vi "PS-OCTA-OCE-autofocus.vi"() -> ()   [LabVIEW 2024] (continued)
  T20 = cluster{"AcqCursorList":T9, "RecalFringePhaseFit_Inv":dbl[][], "RawDualBackgroundArray":i16[][], "RawSingleBackgroundArray":i16[][], "RawRecalFringeArray":i16[][], "RecalFringePhaseFit":dbl[][], "SingleBackground":i16[], "DualBackground":i16[], "image crop start":i32, "cut_level_low":dbl, "cut_level_high":dbl, "Raw1mmFringeArray":i16[][], "img_bckg_offset":i32, "img_bckg_length":i32, "DVV":i16[][], "DVV_shift":i32, "disp_coef":dbl}[]
  T21 = typedef "imagedata.ctl" = cluster{"image type":i32, "image depth":i32, "image":u8[], "mask":u8[], "colors":u32[], "Rectangle":cluster{"left":i16, "top":i16, "right":i16, "bottom":i16}}
  T22 = cluster{"n_f to c. trig":i32, "c. trig length":i32, "c. trig interval":i32, "n_c. trig":i32}
  T23 = cluster{dbl, i32, "cut_level_high":dbl, "cut_level_low":dbl, "offset":i32, "length":i32, "crop start":i32, i32}
  T24 = cluster{"Robot Vel":dbl, "Robot Acc":dbl, "Z-tolerance (mm)":dbl, "Angle tolerance (deg)":dbl, i32, "Radius (mm)":dbl, "Angle End (deg)":dbl, "Number of points":i32, bool, "Z height (pixel)":dbl, "X (mm)":dbl, "Y (mm) ":dbl, "Apply Offset":bool, "Angle Start (deg)":dbl, "N OCT":i32}
  T25 = cluster{"Autofocus":bool, "Freedrive":bool, "Next point":bool, "Previous point":bool, "Home":bool, "Reset":bool, "Start Full Protocol":bool, "3D preview":bool, "Robot ON/OFF":bool, "Cancel Button":bool, "scan_flip_state":bool, "Robot_control":bool, "OCT_control":bool, "OCTA_control":bool, "OCE_control":bool}
  T26 = cluster{"message":string, "angle":dbl, "circle_state":dbl, "scan_trigger":bool, "apply_config":bool, "end_state":bool, "scan_3d":bool, "full_scan":bool, "robot_mode":bool, "oct_mode":bool, "octa_mode":bool, "oce_mode":bool}
  T27 = typedef "ORS_Parameter_Cluster_v8.ctl" = cluster{"file version":u32, "data set dimension":u16, "description":string, "sampling_rate":dbl, "samples_per_line":dbl, "vert_range":dbl, "various params":string, "image samples per line":i32, "image height (crop)":i32, "CPI frequency per mm":dbl, "Peak samp pos\n1mm (Michels)":i32, "n_channel":i32, "Buffer factor":i32, "Per Channel Params":T8, "Galvo":T5, "n_bit":enum16{"8bit", "16bit"}, "timestamp":string}
  T28 = cluster{"samples/line 3d":dbl, "n_lines":i32, "cut_level_high":dbl, "cut_level_low":dbl, "offset":i32, "length":i32, "crop start":i32, "image height":i32}
diagram:
  w10 = T6 {"shutter1"="", "shutter2"="", "Galvo"={"x mirror"="", "y mirror"="", "trig out"="", "x mirror task"="", "y mirror task"="", "trig out task"="", "n_axis"=0, "params"={"n_lines"=0, "n_frames"=0, "force to zero"=FALSE, "Triggers_per_sweep"=0.0, "X center"=0.0, "X span"=0.0, "Y center"=0.0, "Y span"=0.0, "flyb.lines"=0, "n_triggers"=0, "mode"=0, "offset"=0.0, "galvo phase"=0, "span factor"=0.0, "Custom trig."={"n_f to c. trig"=0, "c. trig length"=0, "c. trig interval"=0, "n_c. trig"=0}, "f_per_pos"=0, "n_dataset"=0, "flyback fr"=0}, "acq trig out"="", "acq trig out task"="", "sample array X"=[], "sample array Y"=[], "custom trig out"="", "custom trig out task"="", "FDML-box"="", "ACQ/Galvo"=enum."ADC/FDML", "acq trig out an task"="", "acq trig out an"="", "Galvo Trig input"="", "Galvo Clk input"="", "sample array Acq trig out an"=[]}, "n_bit"=enum."16bit", "diode mon"="", "Misc_I/O"=enum."None"}  # instrument cluster
  w6 = T7 {"Data source"=enum."AlazarTec", "Sample Rate"=0.0, "n_channel"=1, "At9462 # samples"=1024, "image height (crop)"=512, "B scan offset (sps)"=0.0, "window"=0, "OCT data dir"=path "", "3d file name"="", "Description"="", "Galvo params only for file storage"={"n_lines"=0, "n_frames"=0, "force to zero"=FALSE, "Triggers_per_sweep"=0.0, "X center"=0.0, "X span"=0.0, "Y center"=0.0, "Y span"=0.0, "flyb.lines"=0, "n_triggers"=0, "mode"=0, "offset"=0.0, "galvo phase"=0, "span factor"=0.0, "Custom trig."={"n_f to c. trig"=0, "c. trig length"=0, "c. trig interval"=0, "n_c. trig"=0}, "f_per_pos"=0, "n_dataset"=0, "flyback fr"=0}, "Per Channel Params"=[{"AcqCursorList"=[], "RecalFringePhaseFit_Inv"=[], "RawDualBackgroundArray"=[], "RawSingleBackgroundArray"=[], "RawRecalFringeArray"=[], "RecalFringePhaseFit"=[], "SingleBackground"=[], "DualBackground"=[], "image crop start"=0, "cut_level_low"=70.0, "cut_level_high"=110.0, "Raw1mmFringeArray"=[], "img_bckg_offset"=0, "img_bckg_length"=20, "DVV"=[], "DVV_shift"=20, "disp_coef"=0.0}], "file version"=8, "do_dual_card"=FALSE, "ATS_clock"={"Source"=2, "Sample Rate"=48, "Edge"=0, "Rate Ext Ref"=400000000, "Trigger Delay"=100, "Rate Int Ref"=450}, "ATS_clock 2"={"Source"=8, "Sample Rate"=48, "Edge"=0, "Rate Ext Ref"=400000000, "Trigger Delay"=0, "Rate Int Ref"=500}, "DES"=FALSE, "digi_trig"=TRUE, "Ch. Select"=[TRUE, TRUE, FALSE, FALSE, FALSE, FALSE, FALSE, FALSE], "Override Ch."=[FALSE, FALSE, FALSE, FALSE, FALSE, FALSE, FALSE, FALSE], "DoInterp"=TRUE, "EnableDVV"=FALSE, "bufferCount"=128, "dispcoef"=0.0, "AO.type"=12590, "Disable Bck"=[FALSE, FALSE, FALSE, FALSE, FALSE, FALSE, FALSE, FALSE], "PhaseCompVector"=array[2304 elements], "DoDispComp"=FALSE, "Load Insight?"=FALSE, "ChannelDisp"=1, "Zoom Factor"=0.0, "FFT Down Sample"=1, "cut_level_high"=127.0, "cut_level_low"=40.0, "Channel"=3, "IgnoreBadClk"=FALSE, "Good_Clock"=2.65e-06, "Bad_Clock"=2.05e-06}  # General state cluster
  # "command array cmds"
  # "cmds"
  # "instrument cluster - instr"
  n1 = local write "Roll-off"(dbl[][] [] ("Roll-off")) -> ()
  n2 = local write "Roll-off_RawData"(i32[][] [] ("Roll-off")) -> ()
  n3 = call <vilib>:"Application Directory.vi"() -> ("Application Directory"=w4:path)
  n4 = Build Path(base path=w4, name or relative path="Custom state file") -> (appended path=w2:path)
  n5 = call "serial_read_write.vi"("Enable Delayline"="Enable Delayline", "VISA Refnum in"="VISA resource name") -> ()  [unwired: 10 in]
  n6 = Build Array("ConfigAndDisplay") -> (w12:string[])
  n7 = case shown="True" "LoadConfig?" {
    tunnel: w12 -> [w14 w15]
    tunnel: [w14 w17] -> w11
    frame False {
    }
    frame True {
      n8 = Build Array (concatenate)("LoadDefaultState", w15) -> (w17:string[])
    }
  }
  n9 = stacked-sequence {
    seq-local: [w19 _ _] -> [_ w64 w1997]
    tunnel: w6 -> [_ w63 _]
    tunnel: w11 -> [_ w62 _]
    tunnel: [_ w61 _] -> _
    tunnel: w2 -> [_ w60 _]
    tunnel: w10 -> [w21 w58 _]
    tunnel: [_ w59 _] -> _
    frame #0 {
      w18 = enum16{"8bit", "16bit"}."16bit"  # n_bit
      # "INIT\nsystem initialization"
      n10 = Bundle By Name(cluster=w21, "n_bit"=w18) -> (w20:T6)
      n11 = flat-sequence {
        tunnel: w20 -> [w40]
        tunnel: [w37] -> w19
        frame #0 {
          w23 = TRUE ("Apply Acq Config")
          w39 = "(none)" ("Time of background capture")
          # "Misc I/O for shutters & PD monitor"
          # "acq trig for ADC card + Galvo control"
          n12 = local write "exit"(FALSE ("exit")) -> ()
          n13 = local write "Start 3D scan"(FALSE) -> ()
          n14 = local write "Apply Config"(w23) -> ()
          n15 = local write "Apply Acq Config"(w23) -> ()
          n16 = case shown="\"NI_DAQ\"" "Misc_I/O" {
            tunnel: [_ w53 _] -> w42
            tunnel: [_ w52 _] -> w41
            tunnel: [_ w49 _] -> w35
            tunnel: [enum16{"FDML", "NI_DAQ", "None"}."FDML" ("Misc_I/O") enum16{"FDML", "NI_DAQ", "None"}."NI_DAQ" ("Misc_I/O") enum16{"FDML", "NI_DAQ", "None"}."None" ("Misc_I/O")] -> w33
            frame "FDML", Default {
            }
            frame "NI_DAQ" {
              n17 = Build Array("diode monitor +", "diode monitor -") -> (w45:tag[])
              n18 = call <vilib>:"DAQmx Flatten Channel String.vi"("names in"=w45) -> ("names out"=w46:string)  [unwired: 13 in, 1 out]
              n19 = call-poly <vilib>:"DAQmx Create Virtual Channel.vi"("physical channels"=w46) -> ("task out"=w49:refnum<k21>)  [unwired: 13 in, 1 out]
              n20 = call-poly <vilib>:"DAQmx Create Virtual Channel.vi"("lines"="shutter1") -> ("task out"=w53:refnum<k21>)  [unwired: 13 in, 1 out]
              n21 = call-poly <vilib>:"DAQmx Create Virtual Channel.vi"("lines"="shutter2") -> ("task out"=w52:refnum<k21>)  [unwired: 13 in, 1 out]
            }
            frame "None" {
            }
          }
          n22 = local write "Time of last RecalFringes"(w39) -> ()
          n23 = local write "Time of background capture"(w39) -> ()
          n24 = local write "OpModeTab"(enum32{"Config", "Img:Preview"}."Config" ("OpModeTab")) -> ()
          n25 = call "ORS_GalvoInit2_uw.vi"("acq trig out"=tag "Dev1/port0/line4", "custom trig out"=tag "Dev1/port0/line7", "Galvo Clk input"=tag "/Dev1/PFI0", "trig out"=tag "Dev1/port0/line2" ("trig AND out"), "y mirror"=tag "Dev1/ao1", "x mirror"=tag "Dev1/ao0") -> ("Galvo out"=w25:T5)  [unwired: 4 in, 1 out]
          n26 = Bundle By Name(cluster=w25, "ACQ/Galvo"=enum32{"ADC/FDML", "NI_DAQ", "ADC"}."NI_DAQ") -> (w36:T5)
          n27 = Bundle By Name(cluster=w40, "diode mon"=w35, "Galvo"=w36, "shutter1"=w42, "shutter2"=w41, "Misc_I/O"=w33) -> (w37:T6)
        }
      }
    }
    frame #1 {
      w57 = 0  # n_lines
      # "MAIN"
      n28 = feedback #1() -> (w55:u8[][])  [unwired: 1 in]
      n29 = while {
        shift-right: [w87] -> w61
        shift-left: w63 -> [w88]
        shift-right: [w79] -> w59
        shift-left: w64 -> [w93]
        shift-right: [w86] -> _
        shift-left: w62 -> [w68]
        tunnel: w60 -> [w85]
        shift-right: [w84] -> _
        shift-left: _ -> [w77]
        shift-right: [w83] -> _
        shift-left: w57 -> [w82]
        shift-right: [w81] -> _
        shift-left: _ -> [w80]
        shift-right: [w79] -> _
        shift-left: _ -> [w78]
        shift-right: [w76] -> _
        shift-left: _ -> [w75]
        tunnel: w58 -> [w74]
        shift-right: [w72] -> _
        shift-left: _ -> [w71]
        shift-right: [w69] -> _
        shift-left: w55 -> [w70]
        tunnel: [u8[][] []] -> w56
        shift-right: [w65] -> _
        shift-left: _ -> [w66]
        i -> [w89]
        stop <- w73 stop-if-true
        # "skip"
        # "instr"
        # "raw"
        # "state"
        # "instr"
        # "cmds"
        # "samples per line"
        # "number of lines"
        # "This is the main program loop."
        n30 = case shown="\"Img:Preview\"" "OpModeTab" {
          tunnel: w93 -> [w101 w894]
          tunnel: [w100 w871] -> w90
          tunnel: w88 -> [w99 w895]
          tunnel: [w98 w893] -> w87
          tunnel: [w97 w892] -> w79
          tunnel: w68 -> [w96 w890]
          tunnel: [w95 w891] -> w86
          tunnel: w85 -> [w94 _]
          tunnel: [_ w889] -> w84
          tunnel: w77 -> [_ w888]
          tunnel: [_ w887] -> w83
          tunnel: w82 -> [_ w886]
          tunnel: [_ w885] -> w81
          tunnel: w80 -> [_ w884]
          tunnel: w78 -> [_ w883]
          tunnel: w77 -> [_ w882]
          tunnel: [_ w881] -> w76
          tunnel: w75 -> [_ w880]
          tunnel: w74 -> [_ w879]
          tunnel: [_ w878] -> w72
          tunnel: w71 -> [_ w877]
          tunnel: w70 -> [_ w876]
          tunnel: [_ w875] -> w69
          tunnel: w66 -> [_ w874]
          tunnel: [_ w873] -> w65
          frame "Config", Default {
            # "Config Tab"
            n31 = stacked-sequence {
              seq-local: [w114 _] -> [_ w215]
              seq-local: [w110 _] -> [_ w208]
              seq-local: [w112 _] -> [_ w213]
              seq-local: [w111 _] -> [_ w210]
              tunnel: w101 -> [w103 _]
              tunnel: [w122 _] -> w100
              tunnel: w99 -> [w108 _]
              tunnel: [_ w214] -> w98
              tunnel: [_ w209] -> w97
              tunnel: w96 -> [w117 _]
              tunnel: [_ w212] -> w95
              tunnel: w94 -> [_ w211]
              frame #0 {
                n32 = Unbundle By Name(w108) -> ("Per Channel Params"=w107:T8)
                n33 = Unbundle By Name(w103) -> ("Misc_I/O"=w102:enum16{"FDML", "NI_DAQ", "None"})
                n34 = property on="GageCursorList" class="WFGraph (strict)"() -> ("CrsrList"=w105:T9)  [unwired: 2 in, 2 out]
                n35 = for {
                  tunnel: w107 -> [w137] mode=indexing
                  tunnel: [w135] -> w106 mode=indexing
                  tunnel: w105 -> [w136]
                  n36 = Bundle By Name(cluster=w137, "AcqCursorList"=w136) -> (w135:T13)
                }
                n37 = case shown="\"NI_DAQ\"" w102 {
                  tunnel: "Override shutter 1" -> [_ w130]
                  tunnel: "Override shutter 2" -> [_ w129]
                  tunnel: w103 -> [_ w128]
                  frame "FDML", Default {
                  }
                  frame "NI_DAQ" {
                    n38 = Unbundle By Name(w128) -> ("shutter2"=w132:refnum<k21>)
                    n39 = Unbundle By Name(w128) -> ("shutter1"=w134:refnum<k21>)
                    n40 = call-poly <vilib>:"DAQmx Write.vi"("task/channels in"=w134, "auto start"=TRUE, "data"=w130) -> ()  [unwired: 10 in, 3 out]
                    n41 = call-poly <vilib>:"DAQmx Write.vi"("task/channels in"=w132, "auto start"=TRUE, "data"=w129) -> ()  [unwired: 10 in, 3 out]
                  }
                }
                n42 = local read "NumCh"() -> (w104:i32)
                n43 = Bundle By Name(cluster=w108, "Per Channel Params"=w106, "n_channel"=w104) -> (w109:T7)
                n44 = Empty Array?(array=w117) -> (empty?=w118:bool)
                n45 = Not(x=w118) -> (.not. x?=w119:bool)
                n46 = Or(x="Free running", y=w119) -> (x .or. y?=w124:bool)
                n47 = Select(t=0, s=w124, f=-1) -> (s? t:f=w127:i32)
                n48 = event shown="[11] \"exit\": Mouse Down;  \"exit\": Key Down" {
                  selector: _ -> [_ _ _ _ _ _ _ _ _ _ _ _]
                  dyn-events: _ -> [_ _ _ _ _ _ _ _ _ _ _ _]
                  timeout: w127 -> [_ _ _ _ _ _ _ _ _ _ _ _]
                  tunnel: [w138 w150 w155 w161 w166 w171 w174 w179 w185 w200 w202 w205] -> w113
                  tunnel: [_ _ _ _ _ _ _ _ _ _ _ TRUE] -> w122
                  tunnel: w109 -> [w144 w151 w156 w162 w167 w172 w175 w180 w182 w194 w203 w206]
                  tunnel: [w144 w151 w156 w162 w167 w172 w175 w180 w186 w194 w203 w206] -> w110
                  tunnel: w103 -> [w143 w149 w152 w158 w163 w168 w173 w178 w184 w197 w201 w204]
                  tunnel: w117 -> [w139 w150 w154 w159 w164 w170 w174 w179 w185 w200 w202 w205]
                  tunnel: [w143 w149 w152 w158 w163 w168 w173 w178 w184 w195 w201 w204] -> w111
                  event Timeout {
                    # "Event should trigger only on timeout."
                    n49 = event-data() -> ()  [unwired: 1 in, 2 out]
                    n50 = Array Size(array=w139) -> (size(s)=w142:i32)
                    n51 = Decrement(x=w142) -> (x-1=w141:i32)
                    n52 = Index Array(array=w139, index=w141) -> (element=w140:string)
                    n53 = case shown="Default" w140 {
                      tunnel: [w145 w147] -> w138
                      tunnel: w139 -> [w145 w146]
                      frame "ConfigAndDisplay" {
                      }
                      frame Default {
                        n54 = Build Array (concatenate)(w146, "ConfigAndDisplay") -> (w147:string[])
                      }
                    }
                  }
                  event "OpModeTab": Value Change {
                    n55 = event-data() -> ()  [unwired: 1 in, 6 out]
                  }
                  event "Capture Dual Balanced Background": Mouse Down; "Capture Dual Balanced Background": Key Down {
                    n56 = event-data() -> ()  [unwired: 1 in, 5 out]
                    n57 = Build Array (concatenate)(w154, "CaptureDualBalancedBackground") -> (w155:string[])
                  }
                  event "Save state file": Key Down; "Save state file": Mouse Down {
                    w157 = TRUE ("Apply Acq Config")
                    n58 = event-data() -> ()  [unwired: 1 in, 5 out]
                    n59 = local write "Apply Acq Config"(w157) -> ()
                    n60 = local write "Apply Config"(w157) -> ()
                    n61 = Build Array (concatenate)(w159, "SaveState") -> (w161:string[])
                  }
                  event "Load state file": Key Down; "Load state file": Mouse Down {
                    n62 = event-data() -> ()  [unwired: 1 in, 5 out]
                    n63 = Build Array (concatenate)(w164, "LoadState") -> (w166:string[])
                  }
                  event "Acquire Recal Fringes with Mirror": Key Down; "Acquire Recal Fringes with Mirror": Mouse Down {
                    n64 = event-data() -> ()  [unwired: 1 in, 5 out]
                    n65 = Build Array (concatenate)(w170, "RecalFringesMirror") -> (w171:string[])
                  }
                  event "Free running": Value Change {
                    n66 = event-data() -> ()  [unwired: 1 in, 6 out]
                  }
                  event "Re-Scale Y": Value Change {
                    n67 = event-data() -> ()  [unwired: 1 in, 6 out]
                    n68 = property on="Raw captured photodiode data" class="WFGraph (strict)"("YScale.ScaleFit"=u8 1 ("Y Scale.Scale Fit")) -> ()  [unwired: 2 in, 2 out]
                    n69 = local write "Re-Scale Y"(FALSE ("Re-Scale Y")) -> ()
                  }
                  event "Reset Dual Balanced Background": Key Down; "Reset Dual Balanced Background": Mouse Down {
                    n70 = event-data() -> ()  [unwired: 1 in, 5 out]
                    n71 = Unbundle By Name(w182) -> ("Per Channel Params"=w183:T8)
                    n72 = for {
                      tunnel: w183 -> [w187] mode=indexing
                      tunnel: [w188] -> w181 mode=indexing
                      n73 = Unbundle By Name(w187) -> ("DualBackground"=w191:i16[])
                      n74 = Multiply(x=0 ("y"), y=w191) -> (x*y=w190:i32[])
                      n75 = Bundle By Name(cluster=w187, "DualBackground"=w190) -> (w188:T13)
                    }
                    n76 = Bundle By Name(cluster=w182, "Per Channel Params"=w181) -> (w186:T7)
                  }
                  event "XY: Force zero": Value Change {
                    n77 = event-data() -> ("NewVal"=w199:bool)  [unwired: 1 in, 5 out]
                    n78 = local read "digi_trig"() -> (w193:bool)
                    n79 = local read "AO.type"() -> (w192:i32)
                    n80 = Unbundle By Name(w197) -> ("Galvo"=w198:T5)
                    n81 = call "ORS_GalvoForceToZero_uw.vi"("AO.DataXferMech"=w192, "use_digi_trig"=w193, "force to zero"=w199, "Galvo"=w198) -> ("Galvo out"=w196:T5)  [unwired: 6 in, 1 out]
                    n82 = Bundle By Name(cluster=w197, "Galvo"=w196) -> (w195:T6)
                  }
                  event "Override shutter 1", "Override shutter 2": Key Up; "Override shutter 1", "Override shutter 2": Mouse Up {
                    n83 = event-data() -> ()  [unwired: 1 in, 5 out]
                  }
                  event "exit": Mouse Down; "exit": Key Down {
                    # "Event should trigger only on ext."
                    n84 = event-data() -> ()  [unwired: 1 in, 5 out]
                  }
                }
                n85 = Split 1D Array(array=w113, index=1) -> (first subarray=w115:string[], second subarray=w112:string[])
                n86 = Index Array(array=w115) -> (element=w114:string)  [unwired: 1 in]
                "cmd list" <- w117
              }
              frame #1 {
                n87 = case shown="\"1mmFringes\", \"RecalFringes\", \"RecalFringesMirror\"" w215 {
                  selector: w215 -> [_ _ _ _ _ w599]
                  tunnel: w210 -> [w216 w223 w267 w314 w533 w602]
                  tunnel: w208 -> [w218 w224 w263 w309 w523 w601]
                  tunnel: [w218 w224 w239 w311 w524 w600] -> w214
                  tunnel: w213 -> [w217 w225 w268 w313 w529 w597]
                  tunnel: [w217 w225 w268 w312 w530 w598] -> w212
                  tunnel: w211 -> [_ w222 w257 _ _ _]
                  tunnel: [w216 w223 w266 w310 w526 w596] -> w209
                  frame "None", Default {
                    # "This case intentionally does nothing."
                  }
                  frame "SaveState" {
                    n88 = control-ref of="3D_Galvo_Params"() -> (w221:refnum<vi>)
                    n89 = control-ref of="Data Valid Vector"() -> (w220:refnum<vi>)
                    n90 = control-ref of="Save state file"() -> (w219:refnum<vi>)
                    n91 = call "config_save_state.vi"("appended path"=w222, "General state cluster"=w224, "reference 3"=w219, "reference in"=w220, "Cluster in"=w221) -> ()  [unwired: 7 in]
                  }
                  frame "LoadDefaultState", "LoadState" {
                    w260 = T9 [{"Name"="img start", "Color"=16776960, "Style"=8, "Point Style"=13, "Name Visible"=FALSE, "Allow Drag"=TRUE, "Cursor Mode"=0, "Plot"=0, "Index"=0, "Position"={"X"=0.0, "Y"=0.0}, "X Scale"=0, "Y Scale"=0, "Watch Plots"=[], "Watch All Plots"=FALSE, "Plot Area"=0, "Label Offset"={"X"=0.0, "Y"=2937.5}}, {"Name"="img stop", "Color"=16776960, "Style"=8, "Point Style"=13, "Name Visible"=FALSE, "Allow Drag"=TRUE, "Cursor Mode"=0, "Plot"=0, "Index"=0, "Position"={"X"=1000.0, "Y"=0.0}, "X Scale"=0, "Y Scale"=0, "Watch Plots"=[], "Watch All Plots"=FALSE, "Plot Area"=0, "Label Offset"={"X"=3.6556291390728575, "Y"=2937.5}}, {"Name"="recal start", "Color"=16711680, "Style"=8, "Point Style"=13, "Name Visible"=FALSE, "Allow Drag"=TRUE, "Cursor Mode"=0, "Plot"=0, "Index"=0, "Position"={"X"=108.50331125827815, "Y"=0.0}, "X Scale"=0, "Y Scale"=0, "Watch Plots"=[], "Watch All Plots"=FALSE, "Plot Area"=0, "Label Offset"={"X"=0.0, "Y"=2937.5}}, {"Name"="recal stop", "Color"=16711680, "Style"=8, "Point Style"=13, "Name Visible"=FALSE, "Allow Drag"=TRUE, "Cursor Mode"=0, "Plot"=0, "Index"=0, "Position"={"X"=922.2781456953643, "Y"=0.0}, "X Scale"=0, "Y Scale"=0, "Watch Plots"=[], "Watch All Plots"=FALSE, "Plot Area"=0, "Label Offset"={"X"=0.0, "Y"=2937.5}}]  # AcqCursorList_default
                    w280 = T14 4 items=["no dialog", "OK message", "continue or stop message", "OK message + warnings", "continue/stop + warnings"] ("type of dialog (OK msg:1)")
                    # "n_lines is either #lines preview or #lines2d/3d, depending on which one has been last used\n(same for Y span and  Y center, but in almost all cases 2d should have been used before exit)"
                    n92 = local write "Load state file"(FALSE ("Save state file 2")) -> ()
                    n93 = Read from Binary File(5:w263, 9:T10."little-endian" ("byte order (0:big-endian, network order)"), 11:w257) -> (0:w279:errorcluster, 2:w262:T7)  [unwired: 3 in, 2 out]
                    n94 = call <vilib>:"General Error Handler.vi"("type of dialog (OK msg:1)"=w280, "error in (no error)"=w279) -> ("error?"=w264:bool)  [unwired: 9 in, 4 out]
                    n95 = Select(t=w263, s=w264, f=w262) -> (s? t:f=w239:T7)
                    n96 = Unbundle By Name(w239) -> ("Galvo params only for file storage"=w226:T4, "Per Channel Params"=w276:T8, "At9462 # samples"=w277:u32, "image height (crop)"=w271:i32, "B scan offset (sps)"=w270:dbl, "n_channel"=w269:i32, "OCT data dir"=w256:path, "3d file name"=w265:string, "Description"=w255:string, "file version"=→"file version":u32, "do_dual_card"=w254:bool, "ATS_clock"=w252:T1, "ATS_clock 2"=w251:T1, "DES"=w250:bool, "digi_trig"=w253:bool, "Ch. Select"=w243:bool[], "Override Ch."=w242:bool[], "DoInterp"=w244:bool, "EnableDVV"=w245:bool, "bufferCount"=w247:i32, "dispcoef"=w246:dbl, "AO.type"=w248:i32, "Disable Bck"=w249:bool[], "PhaseCompVector"=w241:cdb[], "DoDispComp"=w238:bool, "Load Insight?"=w231:bool, "ChannelDisp"=w236:i32, "Zoom Factor"=w235:sgl, "FFT Down Sample"=w234:i32, "cut_level_high"=w233:dbl, "cut_level_low"=w232:dbl, "Channel"=w230:u32, "IgnoreBadClk"=w229:bool, "Good_Clock"=w228:dbl, "Bad_Clock"=w227:dbl)
                    n97 = case shown="True" w231 {
                      frame False {
                      }
                      frame True {
                        n98 = Not Equal?(x="Data Sample Clk", y="Laser Drive Clk") -> (x != y?=w284:bool)
                        n99 = call <vilib>:"Check if File or Folder Exists.vi"("path"="Insight File Path") -> ("file or folder exists?"=w286:bool, "dup path"=w285:path)  [unwired: 8 in, 1 out]
                        n100 = case shown="True" w286 {
                          tunnel: w285 -> [_ w298]
                          tunnel: w284 -> [_ w295]
                          tunnel: "Data Sample Clk" -> [_ w290]
                          tunnel: "Laser Drive Clk" -> [_ w289]
                          frame False {
                            n101 = One Button Dialog(message="Insight File Path not exist.") -> ()  [unwired: 1 in, 1 out]
                          }
                          frame True {
                            n102 = call "ORS_Insight_Read_Laser_Parameters_from_File.vi"("Save Data Path in"=w298) -> ("Data Valid Vector"=w292:u32[], "Actual Laser Settings Out"=w297:T16)  [unwired: 7 in, 1 out]
                            n103 = Unbundle By Name(w297) -> ("Total Sweep Pts"=→"Total Sweep Pts":i32, "Sample Pts"=w294:u32)
                            n104 = case shown="False" w295 {
                              tunnel: w294 -> [w300 _]
                              tunnel: [w300 w301] -> w293
                              tunnel: w292 -> [w299 w303]
                              tunnel: [w299 w302] -> w291
                              tunnel: w290 -> [_ w305]
                              tunnel: w289 -> [_ w304]
                              frame False {
                              }
                              frame True {
                                n105 = call "Insight_Valid_Vector_Clock_Transform.vi"("Input Valid Vector"=w303, "Laser Drive Clk"=w304, "Data Sample Clk"=w305) -> ("Output Valid Vector"=w302:i32[])  [unwired: 7 in, 1 out]
                                n106 = Array Size(array=w302) -> (size(s)=w301:i32)
                              }
                            }
                            "Sample Pts" <- w293
                            "Data Valid Vector" <- w291
                          }
                        }
                      }
                    }
                    n107 = case shown="True" "loadGalvo" {
                      tunnel: w226 -> [_ w306]
                      frame False {
                      }
                      frame True {
                        n108 = local write "3D_Galvo_Params"(w306) -> ()
                      }
                    }
                    n109 = local write "Channel"(w230) -> ()
                    n110 = local write "NumCh"(w269) -> ()
                    n111 = local write "digi_trig"(w253) -> ()
                    n112 = local write "DoInterp"(w244) -> ()
                    n113 = local write "AO.type"(w248) -> ()
                    n114 = local write "DES"(w250) -> ()
                    n115 = local write "IgnoreBadClk"(w229) -> ()
                    n116 = local write "cut_level_high"(w233) -> ()
                    n117 = local write "cut_level_low"(w232) -> ()
                    n118 = local write "Good_Clock"(w228) -> ()
                    n119 = local write "Bad_Clock"(w227) -> ()
                    n120 = local write "FFT Down Sample"(w234) -> ()
                    n121 = local write "B scan offset"(w270) -> ()
                    n122 = local write "# samples"(w277) -> ()
                    n123 = local write "image height"(w271) -> ()
                    n124 = local write "Description"(w255) -> ()
                    n125 = local write "dual_card"(w254) -> ()
                    n126 = local write "ATS_clock 2"(w251) -> ()
                    n127 = local write "Ch. Select"(w243) -> ()
                    n128 = local write "Override Ch."(w242) -> ()
                    n129 = local write "Enable DVV?"(w245) -> ()
                    n130 = local write "bufferCount"(w247) -> ()
                    n131 = local write "Dispersion coef"(w246) -> ()
                    n132 = local write "Disable Bck"(w249) -> ()
                    n133 = local write "PhaseCompVector"(w241) -> ()
                    n134 = local write "DoDispComp"(w238) -> ()
                    n135 = local write "Load Insight?"(w231) -> ()
                    n136 = local write "ChannelDisp"(w236) -> ()
                    n137 = local write "OCT Zoom"(w235) -> ()
                    n138 = local write "OCT PATH"(w256) -> ()
                    n139 = local write "OCT NAME"(w265) -> ()
                    n140 = local write "ATS_clock"(w252) -> ()
                    n141 = Index Array(array=w276) -> (element=w275:T13)  [unwired: 1 in]
                    n142 = Unbundle By Name(w275) -> ("AcqCursorList"=w259:T9, "image crop start"=w274:i32, "cut_level_low"=w273:dbl, "cut_level_high"=w272:dbl)
                    n143 = Bundle By Name(cluster=w267, "Galvo.params"=w226) -> (w266:T6)
                    n144 = Empty Array?(array=w259) -> (empty?=w261:bool)
                    n145 = Select(t=w260, s=w261, f=w259) -> (s? t:f=w258:T9)
                    n146 = property on="CursorList" class="WFGraph (strict)"("CrsrList"=w258) -> ()  [unwired: 2 in, 2 out]
                    n147 = local write "crop start"(w274) -> ()
                    n148 = local write "cut_level_low"(w273) -> ()
                    n149 = local write "cut_level_high"(w272) -> ()
                  }
                  frame "ConfigAndDisplay" {
                    n150 = Unbundle By Name(w309) -> ("Per Channel Params"=w308:T8)
                    n151 = Index Array(array=w308) -> (element=w307:T13)  [unwired: 1 in]
                    n152 = stacked-sequence {
                      seq-local: [w348 _] -> [_ w473]
                      seq-local: [w322 _] -> [_ w471]
                      tunnel: w314 -> [w351 _]
                      tunnel: w309 -> [w349 _]
                      tunnel: w313 -> [w350 _]
                      tunnel: [w350 _] -> w312
                      tunnel: [_ w473] -> w311
                      tunnel: [w347 _] -> w310
                      tunnel: w307 -> [_ _]
                      frame #0 {
                        n153 = Unbundle By Name(w351) -> ("Galvo"=w321:T5)
                        n154 = local write "Apply Config"(TRUE) -> ()
                        n155 = case shown="True" "dual_card" {
                          tunnel: "ATS_clock" -> [w439 w443]
                          tunnel: [w438 w441] -> w319
                          tunnel: [u32[] [1] u32[] [1, 2]] -> w318
                          frame False {
                            n156 = Build Array(w439) -> (w438:T17)
                          }
                          frame True {
                            n157 = Build Array(w443, "ATS_clock 2") -> (w441:T17)
                          }
                        }
                        n158 = Unbundle By Name(w321) -> ("ACQ/Galvo"=w341:enum16{"ADC/FDML", "NI_DAQ", "ADC"})
                        n159 = Unbundle By Name("ATS_clock") -> ("Source"=w342:u32)
                        n160 = case shown="Default" w342 {
                          tunnel: "ATS_clock" -> [w447 w449 w451 _]
                          tunnel: [w445 w448 w450 w452] -> w344
                          tunnel: w341 -> [_ _ _ w453]
                          frame 1 {
                            n161 = Unbundle By Name(w447) -> ("Source"=w444:u32)
                            n162 = Multiply(x=w444, y=1000.0 ("Sample Rate")) -> (x*y=w445:dbl)
                          }
                          frame 7 {
                            n163 = Unbundle By Name(w449) -> ("Rate Ext Ref"=w448:u32)
                          }
                          frame 8 {
                            n164 = Unbundle By Name(w451) -> ("Rate Int Ref"=w450:u32)
                          }
                          frame Default {
                            n165 = case shown="\"ADC/FDML\", Default" w453 {
                              tunnel: [w454 "ext sample_rate"] -> w452
                              frame "ADC/FDML", Default {
                                # "To do:\nread from FDML laser"
                                n166 = local read "ext sample_rate"() -> (w454:dbl)
                              }
                              frame "NI_DAQ", "ADC" {
                                # "get sample rate from FDML"
                              }
                            }
                          }
                        }
                        "sample rate (S/s)" <- w344
                        n167 = property on="Raw captured photodiode data" class="WFGraph (strict)"() -> ("CrsrList"=w338:T9)  [unwired: 2 in, 2 out]
                        n168 = stacked-sequence {
                          seq-local: [w353 _ _ _] -> [_ w360 _ _]
                          seq-local: [w352 _ _ _] -> [_ w355 _ _]
                          tunnel: "# samples" -> [w353 _ _ _]
                          tunnel: [w354 _ _ _] -> w345
                          tunnel: w319 -> [_ w361 _ _]
                          tunnel: w321 -> [_ w358 _ _]
                          tunnel: w318 -> [_ w357 _ _]
                          tunnel: [_ w356 _ _] -> w316
                          tunnel: [_ _ w408 _] -> w322
                          tunnel: "# samples" -> [_ _ w411 _]
                          tunnel: [_ _ _ w436] -> w343
                          frame #0 {
                            n169 = local read "Laser Trigger"() -> (w352:bool)
                            n170 = Tick Count (ms)() -> (millisecond timer value=w354:u32)
                          }
                          frame #1 {
                            n171 = local read "Apply Acq Config"() -> (w359:bool)
                            n172 = case shown="True" w359 {
                              tunnel: w361 -> [_ w383]
                              tunnel: w360 -> [_ w373]
                              tunnel: w358 -> [w363 w380]
                              tunnel: [w363 w377] -> w356
                              tunnel: w357 -> [_ w371]
                              tunnel: w355 -> [_ w364]
                              frame False {
                                n173 = Wait (ms)(milliseconds to wait=u32 10) -> ()  [unwired: 1 out]
                              }
                              frame True {
                                w368 = 400  # n_triggers
                                n174 = Array Size(array=w371) -> (size(s)=w370:i32)
                                n175 = for {
                                tunnel: w383 -> [w404] mode=indexing
                                tunnel: [w398] -> w375 mode=indexing
                                tunnel: w371 -> [w403] mode=indexing
                                tunnel: w368 -> [_]
                                tunnel: [w402] -> w374
                                tunnel: w373 -> [w399]
                                tunnel: [w388] -> w366
                                tunnel: ["Channel"] -> w365
                                tunnel: w364 -> [w384]
                                (unwired) u32 2048 ("Records Count")
                                n176 = Wait (ms)(milliseconds to wait=u32 10) -> ()  [unwired: 1 out]
                                n177 = call "ORS_AlazarDLLCfg_All.vi"("Bad Clock Duration"="Bad_Clock", "Good Clock Duration"="Good_Clock", "DESmode"="DES", "IgnoreBadClk"="IgnoreBadClk", "ATS_clock"=w404, "bufferCount"="bufferCount", "Channel"="Channel", "Range"="AT_Range", "System ID"=w403) -> ("error out"=w397:errorcluster, "ATSHandle"=w400:u32)  [unwired: 1 in]
                                n178 = call "ORS_AlazarDLLAcq_Prepare.vi"("Lamda Trigger?"=w384, "Channel"="Channel", "Records Per Buffer"=u32 12288, "error in (no error)"=w397, "Records Count"=u32 2147483647, "Record length"=w399, "ATSHandle"=w400) -> ("error out"=w396:errorcluster, "Samps Per Buffer"=w402:u32, "ATSHandle_out"=w401:u32)  [unwired: 2 in]
                                n179 = call "ORS_AlazarDLLAcq_Start.vi"("error in (no error)"=w396, "ATSHandle"=w401) -> ("error out"=w388:errorcluster, "ATSHandle_out"=w398:u32)  [unwired: 8 in]
                                }
                                "ATSHandle" <- w375
                                "Samps Per Buffer Config" <- w374
                                n180 = call "ORS_GalvoConfig1D_uw.vi"("Force to zero"=FALSE, "use_digi_trig"="digi_trig", "n_triggers"=w368, "Galvo"=w380) -> ("Galvo out"=w381:T5)  [unwired: 6 in, 1 out]
                                n181 = call "ORS_GalvoPrepareScan_uw-1kp.vi"("use_digi_trig"="digi_trig", "AO.DataXferMech"="AO.type", "Galvo"=w381) -> ("Galvo out"=w379:T5)  [unwired: 5 in, 3 out]
                                n182 = call "ORS_GalvoStartScan.vi"("Galvo"=w379) -> ("Galvo out"=w378:T5)  [unwired: 9 in, 1 out]
                                n183 = call "ORS_GalvoCleanupScan.vi"("Galvo"=w378) -> ("Galvo out"=w377:T5)  [unwired: 9 in, 1 out]
                                n184 = call <vilib>:"Simple Error Handler.vi"("error in (no error)"=w366) -> ()  [unwired: 4 in, 5 out]
                                n185 = case shown="3" w365 {
                                tunnel: [u8 1 u8 1 u8 2] -> w372
                                frame 1, Default {
                                }
                                frame 2 {
                                }
                                frame 3 {
                                }
                                }
                                n186 = Multiply(x=w372, y=w370) -> (x*y=→"NumCh":i32)
                              }
                            }
                          }
                          frame #2 {
                            # "Wait for acquisition"
                            n187 = local read "do_highpass"() -> (w414:bool)
                            n188 = local read "Samps Per Buffer Config"() -> (w417:u32)
                            n189 = local read "ATSHandle"() -> (w418:u32[])
                            n190 = Array Size(array=w418) -> (size(s)=w415:i32)
                            n191 = local read "NumCh"() -> (w423:i32)
                            n192 = Multiply(x=w417, y=w415) -> (x*y=w416:u32)
                            n193 = call "ORS_AlazarDLLAcq_XferLatestFrame.vi"("SamplesPerBuffer"=w417, "ATSHandle"=w418) -> ("Return Code"=w421:u32, "Buffer"=w422:u16[])  [unwired: 7 in, 1 out]
                            "Cfg Return" <- w421
                            n194 = Divide(x=w416, y=w423) -> (x/y=w424:dbl)
                            n195 = Not Equal?(x=w421, y=u32 512) -> (x != y?=w419:bool)
                            n196 = local write "Apply Acq Config"(w419) -> ()
                            n197 = Reshape Array(w422, w423, w424) -> (w412:u16[][])
                            n198 = Array Subset(array=w412, length (col)=w411) -> (w413:u16[][])  [unwired: 3 in]
                            n199 = for {
                              tunnel: w414 -> [w427]
                              tunnel: w413 -> [w426] mode=indexing
                              tunnel: [w425] -> w409 mode=indexing
                              n200 = case shown="False" w427 {
                                tunnel: w426 -> [w429 w431]
                                tunnel: [w428 w433] -> w425
                                frame False {
                                n201 = To Double Precision Float(number=w429) -> (double precision float=w428:dbl[])
                                }
                                frame True {
                                n202 = To Double Precision Float(number=w431) -> (double precision float=w430:dbl[])
                                n203 = local read "passband"() -> (w434:i32)
                                n204 = call "FFT_filter.vi"("stopband_ratio"=0.05, "passband"=w434, "Input"=w430) -> ("Spectrum_Window"=w432:dbl[][], "Results"=w433:dbl[])  [unwired: 7 in]
                                n205 = local write "Spectrum_Window"(w432) -> ()
                                }
                              }
                            }
                            n206 = Subtract(x=w409, y=32768.0) -> (x-y=w408:dbl[][])
                          }
                          frame #3 {
                            n207 = Tick Count (ms)() -> (millisecond timer value=w436:u32)
                          }
                        }
                        n208 = Decrement(x="# samples") -> (x-1=w325:u32)
                        n209 = Subtract(x=w325, y="Cut_end") -> (x-y=w324:u32)
                        n210 = Index Array(array=w338, index #1=0 ("index")) -> (element #1=w336:T18, element #2=w334:T18, element #3=w331:T18, element #4=w330:T18)  [unwired: 3 in]
                        n211 = Bundle By Name(cluster=w336, "Position.X"="Cut_start") -> (w335:T18)
                        n212 = Bundle By Name(cluster=w334, "Position.X"=w324) -> (w333:T18)
                        n213 = Bundle By Name(cluster=w331, "Position.X"="Cut_start") -> (w328:T18)
                        n214 = Bundle By Name(cluster=w330, "Position.X"=w324) -> (w327:T18)
                        n215 = Build Array(w335, w333, w328, w327) -> (w332:T19)
                        n216 = Replace Array Subset(array=w338, new element=w332, index=0) -> (w339:T9)
                        n217 = property on="Raw captured photodiode data" class="WFGraph (strict)"("CrsrList"=w339) -> ()  [unwired: 2 in, 2 out]
                        n218 = Bundle By Name(cluster=w349, "Sample Rate"=w344, "At9462 # samples"="# samples") -> (w348:T7)
                        n219 = Subtract(x=w343, y=w345) -> (x-y=→"t_config":u32)
                        n220 = Bundle By Name(cluster=w351, "Galvo"=w316) -> (w347:T6)
                      }
                      frame #1 {
                        n221 = Unbundle By Name(w473) -> ("Sample Rate"=w474:dbl, "Per Channel Params"=w472:T8)
                        n222 = for {
                          tunnel: w474 -> [w514]
                          tunnel: [w507] -> w470 mode=concatenating
                          tunnel: w472 -> [w509] mode=indexing
                          tunnel: w471 -> [w492] mode=indexing
                          tunnel: [w487] -> w459 mode=concatenating
                          tunnel: [w486] -> w465 mode=concatenating
                          tunnel: [w488] -> w463 mode=concatenating
                          n223 = local read "PhaseCompVector"() -> (w485:cdb[])
                          n224 = local read "DoDispComp"() -> (w483:bool)
                          n225 = Unbundle By Name(w509) -> ("DualBackground"=w510:i16[], "RecalFringePhaseFit"=w513:dbl[][], "RecalFringePhaseFit_Inv"=w512:dbl[][], "AcqCursorList"=w511:T9)
                          n226 = local read "Data Valid Vector"() -> (w497:u32[])
                          n227 = local read "Cut_start"() -> (w493:u32)
                          n228 = local read "# samples"() -> (w491:u32)
                          n229 = local read "DoInterp"() -> (w484:bool)
                          n230 = Array Subset(array=w492, length=w491) -> (w490:dbl[])  [unwired: 1 in]
                          n231 = Index Array(array=w513) -> (element=w500:dbl[])  [unwired: 2 in]
                          n232 = Index Array(array=w512) -> (element=w501:dbl[])  [unwired: 2 in]
                          n233 = Build Array(w500, w501) -> (w489:dbl[][])
                          n234 = call "ORS_ImgQuickRecaForConfig_DVV.vi"("PhaseCompVector"=w485, "RecalFringePhaseFit"=w500, "window parameter"="window parameter", "Offset"=w493, "Data input"=w490, "DualBackground"=w510, "Sample rate"=w514, "Enable DVV?"="Enable DVV?", "Window"="Window", "Cursor List"=w511, "Cursor crop?"="Cursor crop?", "Valid Vector"=w497, "do_interp"=w484, "DVV shift"="DVV shift", "do_disp_comp"=w483, "Log?"="Log?") -> ("graph output"=w487:dbl[], "FFT max"=→"FFT max: Amplitude":dbl, "1lineFringe"=w486:dbl[], "FFT max index"=→"Idx":i32, "DVV waveform"=→"XY Graph":T3, "FFT max freq (MHz)"=→"FFT max: Freq (MHz)":dbl)  [unwired: 5 in, 1 out]
                          n235 = Transpose 2D Array(2D array=w489) -> (transposed array=w488:dbl[][])
                          n236 = Build Array(w486, w510) -> (w508:dbl[][])
                          n237 = Transpose 2D Array(2D array=w508) -> (transposed array=w507:dbl[][])
                        }
                        "FFT/Ch2" <- w459
                        n238 = case shown="True" "Roll-off" {
                          tunnel: [w476 w482] -> w468
                          tunnel: [w475 w480] -> w467
                          tunnel: w459 -> [_ w478]
                          tunnel: w465 -> [_ w477]
                          frame False {
                            n239 = local read "Roll-off_RawData"() -> (w475:dbl[][])
                            n240 = local read "Roll-off"() -> (w476:dbl[][])
                          }
                          frame True {
                            n241 = local read "Roll-off_RawData"() -> (w479:dbl[][])
                            n242 = local read "Roll-off"() -> (w481:dbl[][])
                            n243 = Build Array (concatenate)(w479, w477) -> (w480:dbl[][])
                            n244 = Build Array (concatenate)(w481, w478) -> (w482:dbl[][])
                          }
                        }
                        "Roll-off" <- w468
                        "Roll-off_RawData" <- w467
                        n245 = Transpose 2D Array(2D array=w463) -> (transposed array=w464:dbl[][])
                        n246 = Transpose 2D Array(2D array=w470) -> (transposed array=→"Raw captured photodiode data":dbl[][])
                        n247 = Array Subset(array=w459, index=100, length=1200) -> (w456:dbl[])
                        n248 = local write "Debug: Final phase fit"(w464) -> ()
                        n249 = Array Max & Min(array=w456) -> (max value=w462:dbl)  [unwired: 3 out]
                        "Signal" <- w462
                        n250 = call <vilib>:"Median.vi"("X"=w456) -> ("median"=w461:dbl)  [unwired: 1 out]
                        "NoiseLv" <- w461
                        n251 = Subtract(x=w462, y=w461) -> (x-y=→"SNR":dbl)
                      }
                    }
                  }
                  frame "CaptureDualBalancedBackground" {
                    n252 = To Word Integer(number=w518) -> (16bit integer=w525:i16[][])
                    n253 = Unbundle By Name(w523) -> ("Per Channel Params"=w521:T8)
                    n254 = Index Array(array=w521) -> (element=w517:T13)  [unwired: 1 in]
                    n255 = flat-sequence {
                      tunnel: w533 -> [w559]
                      tunnel: [w559] -> w532
                      tunnel: ["Number of measurements (dual back)"] -> w527
                      tunnel: [w583] -> w531
                      tunnel: [w575] -> w518
                      tunnel: [w577] -> w519
                      tunnel: w532 -> [w581]
                      tunnel: w527 -> [w584]
                      tunnel: [w572] -> w516
                      tunnel: [w569] -> w515
                      tunnel: w531 -> [w586]
                      tunnel: [w586] -> w526
                      frame #0 {
                        w561 = TRUE  # close sample arm
                        n256 = Unbundle By Name(w559) -> ("Misc_I/O"=w558:enum16{"FDML", "NI_DAQ", "None"})
                        n257 = case shown="\"NI_DAQ\"" w558 {
                          tunnel: w561 -> [w566 _]
                          tunnel: w559 -> [w563 _]
                          tunnel: [u32 500 ("Zu wartende ms") u32 0 ("Zu wartende ms")] -> w557
                          frame "NI_DAQ" {
                            n258 = Unbundle By Name(w563) -> ("shutter1"=w564:refnum<k21>)
                            n259 = call-poly <vilib>:"DAQmx Write.vi"("task/channels in"=w564, "auto start"=TRUE, "data"=w566) -> ()  [unwired: 10 in, 3 out]
                          }
                          frame "None", Default {
                          }
                        }
                        n260 = Wait (ms)(milliseconds to wait=w557) -> ()  [unwired: 1 out]
                      }
                      frame #1 {
                        n261 = local read "ATSHandle"() -> (w579:u32[])
                        n262 = local read "# samples"() -> (w569:u32)
                        n263 = local read "digi_trig"() -> (w570:bool)
                        n264 = local read "Channel"() -> (w571:u32)
                        n265 = local read "AO.type"() -> (w568:i32)
                        n266 = local read "NumCh"() -> (w572:i32)
                        n267 = Unbundle By Name(w581) -> ("Galvo"=w580:T5)
                        n268 = call "ORS_Alazar_acquire_multiple_frames_galvo.vi"("AO.DataXferMech"=w568, "Channel"=w571, "Galvo"=w580, "use_digi_trig"=w570, "frame length"=w569, "# frames"=w584, "ATSHandle"=w579) -> ("Averaged Output"=w574:dbl[], "RawOutputs"=w578:i16[][], "Galvo out"=w582:T5)  [unwired: 2 in]
                        n269 = Bundle By Name(cluster=w581, "Galvo"=w582) -> (w583:T6)
                        n270 = Reshape Array(w574, w572, w569) -> (w575:dbl[][])
                        n271 = Array Size(array=w578) -> (size(s)=w576:i32[])
                        n272 = Index Array(array=w576) -> (element=w573:i32)  [unwired: 1 in]
                        n273 = Reshape Array(w578, w572, w573, w569) -> (w577:i16[][][])
                      }
                      frame #2 {
                        w590 = FALSE ("Capture background")
                        w591 = FALSE  # open
                        n274 = Unbundle By Name(w586) -> ("Misc_I/O"=w587:enum16{"FDML", "NI_DAQ", "None"})
                        n275 = local write "Apply Acq Config"(TRUE ("Apply Acq Config")) -> ()
                        n276 = Get Date/Time String(want seconds? (F)=TRUE ("Angabe von Sekunden? (F)")) -> (time string=→"Time of background capture":string)  [unwired: 2 in, 1 out]
                        n277 = local write "Reset Dual Balanced Background"(w590) -> ()
                        n278 = local write "Capture Dual Balanced Background"(w590) -> ()
                        n279 = case shown="\"NI_DAQ\"" w587 {
                          tunnel: w591 -> [w595 _]
                          tunnel: w586 -> [w592 _]
                          frame "NI_DAQ" {
                            n280 = Unbundle By Name(w592) -> ("shutter1"=w593:refnum<k21>)
                            n281 = call-poly <vilib>:"DAQmx Write.vi"("task/channels in"=w593, "auto start"=TRUE, "data"=w595) -> ()  [unwired: 10 in, 3 out]
                          }
                          frame "None", Default {
                          }
                        }
                      }
                    }
                    n282 = Initialize Array(w517, w516) -> (w520:T20)
                    n283 = Build Array (concatenate)(w529, "SaveState") -> (w530:string[])
                    n284 = for {
                      tunnel: w525 -> [w537] mode=indexing
                      tunnel: w519 -> [w544] mode=indexing
                      tunnel: [w543] -> w522 mode=indexing
                      tunnel: w520 -> [w542] mode=indexing
                      tunnel: w515 -> [w534]
                      i -> [w539]
                      n285 = local read "Enable DVV?"() -> (w536:bool)
                      n286 = case shown="True" w536 {
                        tunnel: w537 -> [w545 w552]
                        tunnel: [w545 w551] -> w535
                        tunnel: w534 -> [_ w546]
                        frame False {
                        }
                        frame True {
                          n287 = local read "DVV shift"() -> (w549:i32)
                          n288 = local read "Data Valid Vector"() -> (w550:u32[])
                          n289 = call "ORS_Insight_Reduce_B-scan_Data.vi"("length"=w546, "offset"=0, "Data Valid Vector"=w550, "spl per line"=w546, "DVV shift"=w549, "line Num"=1, "Input"=w552) -> ("Output"=w551:i16[])  [unwired: 4 in]
                        }
                      }
                      n290 = Index Array(array="Disable Bck", index=w539) -> (element=w538:bool)
                      n291 = case shown="True" w538 {
                        tunnel: w535 -> [w553 w556]
                        tunnel: [w553 w555] -> w541
                        frame False {
                        }
                        frame True {
                          n292 = Multiply(x=w556, y=i16 0) -> (x*y=w555:i16[])
                        }
                      }
                      n293 = Bundle By Name(cluster=w542, "RawDualBackgroundArray"=w544, "DualBackground"=w541) -> (w543:T13)
                    }
                    n294 = Bundle By Name(cluster=w523, "Per Channel Params"=w522) -> (w524:T7)
                  }
                  frame "1mmFringes", "RecalFringes", "RecalFringesMirror" {
                    # "raw data"
                    # "# measurements"
                    n295 = stacked-sequence {
                      seq-local: ["Number of measurements" _ _] -> [_ _ _]
                      seq-local: [w609 _ _] -> [_ w647 _]
                      seq-local: [w603 _ _] -> [_ w645 _]
                      tunnel: w602 -> [w606 _ w865]
                      tunnel: [_ w646 _] -> w600
                      tunnel: w601 -> [w609 _ _]
                      tunnel: w599 -> [w610 w644 w864]
                      tunnel: [_ _ w867] -> w598
                      tunnel: w597 -> [_ _ w866]
                      tunnel: [_ _ w865] -> w596
                      frame #0 {
                        n296 = flat-sequence {
                          tunnel: w606 -> [w612]
                          tunnel: "Number of measurements" -> [w633]
                          tunnel: [w628] -> w603
                          tunnel: w605 -> [w632]
                          tunnel: [w631] -> w604
                          tunnel: w610 -> [_]
                          tunnel: w607 -> [w635]
                          frame #0 {
                            # "close sample arm, open recal arm"
                            n297 = Unbundle By Name(w612) -> ("Misc_I/O"=w611:enum16{"FDML", "NI_DAQ", "None"})
                            n298 = case shown="\"NI_DAQ\"" w611 {
                              tunnel: w612 -> [_ w615 _ _]
                              frame Default {
                              }
                              frame "NI_DAQ" {
                                # "close sample arm, open recal arm"
                                n299 = Unbundle By Name(w615) -> ("shutter1"=w614:refnum<k21>)
                                n300 = Unbundle By Name(w615) -> ("shutter2"=w613:refnum<k21>)
                                n301 = Wait (ms)(milliseconds to wait=u32 500 ("Zu wartende ms")) -> ()  [unwired: 1 out]
                                n302 = call-poly <vilib>:"DAQmx Write.vi"("task/channels in"=w613, "auto start"=TRUE, "data"=TRUE) -> ()  [unwired: 10 in, 3 out]
                                n303 = call-poly <vilib>:"DAQmx Write.vi"("task/channels in"=w614, "auto start"=TRUE, "data"=TRUE) -> ()  [unwired: 10 in, 3 out]
                              }
                              frame "None" {
                              }
                              frame "FDML" {
                              }
                            }
                          }
                          frame #1 {
                            n304 = local read "ATSHandle"() -> (w630:u32[])
                            n305 = local read "# samples"() -> (w624:u32)
                            n306 = local read "digi_trig"() -> (w622:bool)
                            n307 = local read "Channel"() -> (w623:u32)
                            n308 = local read "AO.type"() -> (w621:i32)
                            n309 = call "ORS_Alazar_acquire_multiple_frames_galvo.vi"("AO.DataXferMech"=w621, "Channel"=w623, "Galvo"=w632, "use_digi_trig"=w622, "frame length"=w624, "# frames"=w633, "ATSHandle"=w630) -> ("RawOutputs"=w627:i16[][], "Galvo out"=w631:T5)  [unwired: 2 in, 1 out]
                            n310 = Array Size(array=w627) -> (size(s)=w629:i32[])
                            n311 = local read "NumCh"() -> (w626:i32)
                            n312 = Index Array(array=w629) -> (element=w625:i32)  [unwired: 1 in]
                            n313 = Reshape Array(w627, w626, w625, w624) -> (w628:i16[][][])
                          }
                          frame #2 {
                            n314 = Unbundle By Name(w635) -> ("Misc_I/O"=w634:enum16{"FDML", "NI_DAQ", "None"})
                            n315 = Wait (ms)(milliseconds to wait=u32 50 ("Zu wartende ms")) -> ()  [unwired: 1 out]
                            n316 = case shown="\"NI_DAQ\"" w634 {
                              tunnel: w635 -> [_ _ w643]
                              frame "FDML", Default {
                              }
                              frame "None" {
                              }
                              frame "NI_DAQ" {
                                n317 = Unbundle By Name(w643) -> ("shutter2"=w637:refnum<k21>)
                                n318 = Unbundle By Name(w643) -> ("shutter1"=w638:refnum<k21>)
                                n319 = call-poly <vilib>:"DAQmx Write.vi"("task/channels in"=w637, "auto start"=TRUE, "data"=FALSE) -> ()  [unwired: 10 in, 3 out]
                                n320 = call-poly <vilib>:"DAQmx Write.vi"("task/channels in"=w638, "auto start"=TRUE, "data"=FALSE) -> ()  [unwired: 10 in, 3 out]
                              }
                            }
                          }
                        }
                        n321 = Unbundle By Name(w606) -> ("Galvo"=w605:T5)
                        n322 = Bundle By Name(cluster=w606, "Galvo"=w604) -> (w607:T6)
                      }
                      frame #1 {
                        n323 = case shown="\"RecalFringes\", \"RecalFringesMirror\", Default" w644 {
                          tunnel: w647 -> [w653]
                          tunnel: [w655] -> w646
                          tunnel: w645 -> [w654]
                          frame "RecalFringes", "RecalFringesMirror", Default {
                            n324 = Unbundle By Name(w653) -> ("Per Channel Params"=w649:T8, "Sample Rate"=w656:dbl)
                            n325 = local read "# samples"() -> (w652:u32)
                            n326 = for {
                              tunnel: w654 -> [w674] mode=indexing
                              tunnel: w656 -> [w677]
                              tunnel: w649 -> [w670] mode=indexing
                              tunnel: w652 -> [w672]
                              tunnel: [w660] -> w651 mode=concatenating
                              shift-right: [w663] -> w648
                              shift-left: w649 -> [w666]
                              i -> [w664]
                              # "outer loop: channels"
                              n327 = Unbundle By Name(w670) -> ("DualBackground"=w675:i16[])
                              n328 = Unbundle By Name(w670) -> ("AcqCursorList"=w673:T9)
                              n329 = Index Array(array="Ch. Select", index=w664) -> (element=w668:bool)
                              n330 = Index Array(array="Override Ch.", index=w664) -> (element=w665:bool)
                              n331 = for {
                                N: 1 -> [_]
                                tunnel: [w806] -> w676 mode=indexing
                                tunnel: w674 -> [w826]
                                tunnel: w677 -> [w810]
                                tunnel: w675 -> [w813]
                                tunnel: w673 -> [w792]
                                tunnel: w672 -> [w809]
                                tunnel: [w801] -> w661
                                tunnel: [w796] -> w658 mode=indexing
                                tunnel: [w795] -> w657
                                i -> [w815]
                                w828 = 1 items=["nearest", "linear", "spline", "cubic Hermite", "Lagrange"] ("interpolation method")
                                w824 = 1 items=["nächste", "linear", "Spline", "Hermite (kubisch)", "Lagrange"] ("interpolation method")
                                # "inner loop: buffering"
                                n332 = call "ORS_CursorToCropIdx.vi"("index offset"=0, "Cursor List"=w792) -> ("length"=w829:i32, "offset"=w817:i32)  [unwired: 8 in]
                                n333 = Multiply(x=w815, y=w809) -> (x*y=w803:u32)
                                n334 = Add(x=w803, y=w817) -> (x+y=w816:u32)
                                n335 = Reciprocal(x=w810) -> (1/x=w821:dbl)
                                n336 = for {
                                tunnel: w826 -> [w845] mode=indexing
                                tunnel: w813 -> [w843]
                                tunnel: w816 -> [w848]
                                tunnel: w829 -> [w849]
                                tunnel: [w841] -> w812 mode=indexing
                                n337 = Array Subset(array=w845, index=w848, length=w849) -> (w847:i16[])
                                n338 = local read "Enable DVV?"() -> (w846:bool)
                                n339 = case shown="True" w846 {
                                tunnel: w847 -> [w857 w861]
                                tunnel: [w857 w860] -> w844
                                frame False {
                                }
                                frame True {
                                n340 = local read "Data Valid Vector"() -> (w858:u32[])
                                n341 = local read "DVV shift"() -> (w859:i32)
                                n342 = call "ORS_Insight_Reduce_Data_with_Valid-Vector.vi"("Valid Vector"=w858, "DVV shift"=w859, "Raw Data"=w861) -> ("Valid Data"=w860:i16[])  [unwired: 8 in]
                                }
                                }
                                n343 = Subtract(x=w844, y=w843) -> (x-y=w842:i16[])
                                n344 = case shown="True" "do_highpass" {
                                tunnel: w842 -> [w850 w856]
                                tunnel: [w850 w852] -> w841
                                frame False {
                                }
                                frame True {
                                n345 = call "FFT_filter.vi"("stopband_ratio"=0.05, "passband"="passband", "Input"=w856) -> ("Spectrum_Window"=→"Spectrum_Window":dbl[][], "Results"=w851:dbl[])  [unwired: 7 in]
                                n346 = call-poly <vilib>:"Cosine Tapered Window.vi"("X"=w851) -> ("Windowed X"=w852:dbl[])  [unwired: 9 in, 1 out]
                                }
                                }
                                }
                                n347 = call "ORS_CursorToCropIdx.vi"("index offset"=0 ("cursor index offset"), "Cursor List"=w792) -> ("length"=w790:i32, "offset"=w791:i32)  [unwired: 8 in]
                                n348 = Transpose 2D Array(2D array=w812) -> (transposed array=w823:dbl[][])
